vi "Time.String to TimeStamp.vi"(7 "TimeFormat":T1, 11 "Time String In":string) -> (3 "Time Stamp Out":timestamp)   [LabVIEW 2018]
uses:
  Time.Format Selector.ctl
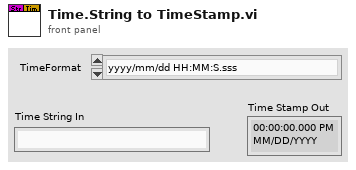
[diagram p1: front panel]
types:
  T1 = typedef "Time.Format Selector.ctl" = enum16{"yyyy/mm/dd HH:MM:S.sss", "yyyy-MM-ddTHH:mm:ss[.mmm]"}
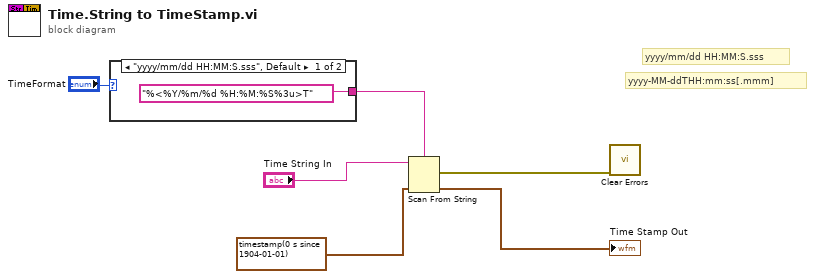
[diagram p0: block diagram]
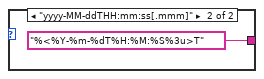
[diagram p2: hidden frame]
diagram:
  # "yyyy/mm/dd HH:MM:S.sss"
  # "yyyy-MM-ddTHH:mm:ss[.mmm]"
  n1 = case shown="\"yyyy/mm/dd HH:MM:S.sss\", Default" "TimeFormat" {
    tunnel: ["%<%Y/%m/%d %H:%M:%S%3u>T" ("time format string (%c)") "%<%Y-%m-%dT%H:%M:%S%3u>T" ("time format string (%c)")] -> w1
    frame "yyyy/mm/dd HH:MM:S.sss", Default {
    }
    frame "yyyy-MM-ddTHH:mm:ss[.mmm]" {
    }
  }
  n2 = Scan From String(format string=w1, input string="Time String In", default 1=timestamp(0 s since 1904-01-01) ("Time Stamp Out")) -> (error out=w3:errorcluster, output 1=→"Time Stamp Out":timestamp)  [unwired: 2 in, 2 out]
  n3 = call <vilib>:"Clear Errors.vi"("error in (no error)"=w3) -> ()  [unwired: 5 in, 2 out]
